vi "time_to_mass.vi"(1 "C1 Data":T3, 3 "C2 Data":T3, 5 "Vairables Cluster":T1, 11 "error in (no error)":errorcluster) -> (12 "C1 Mass Data":T2, 14 "C2 Mass Data":T2, 15 "error out":errorcluster)   [LabVIEW 2023]
uses:
  <vilib>/Waveform/WDTOps.llb/WDT Get Waveform Time Array DBL.vi
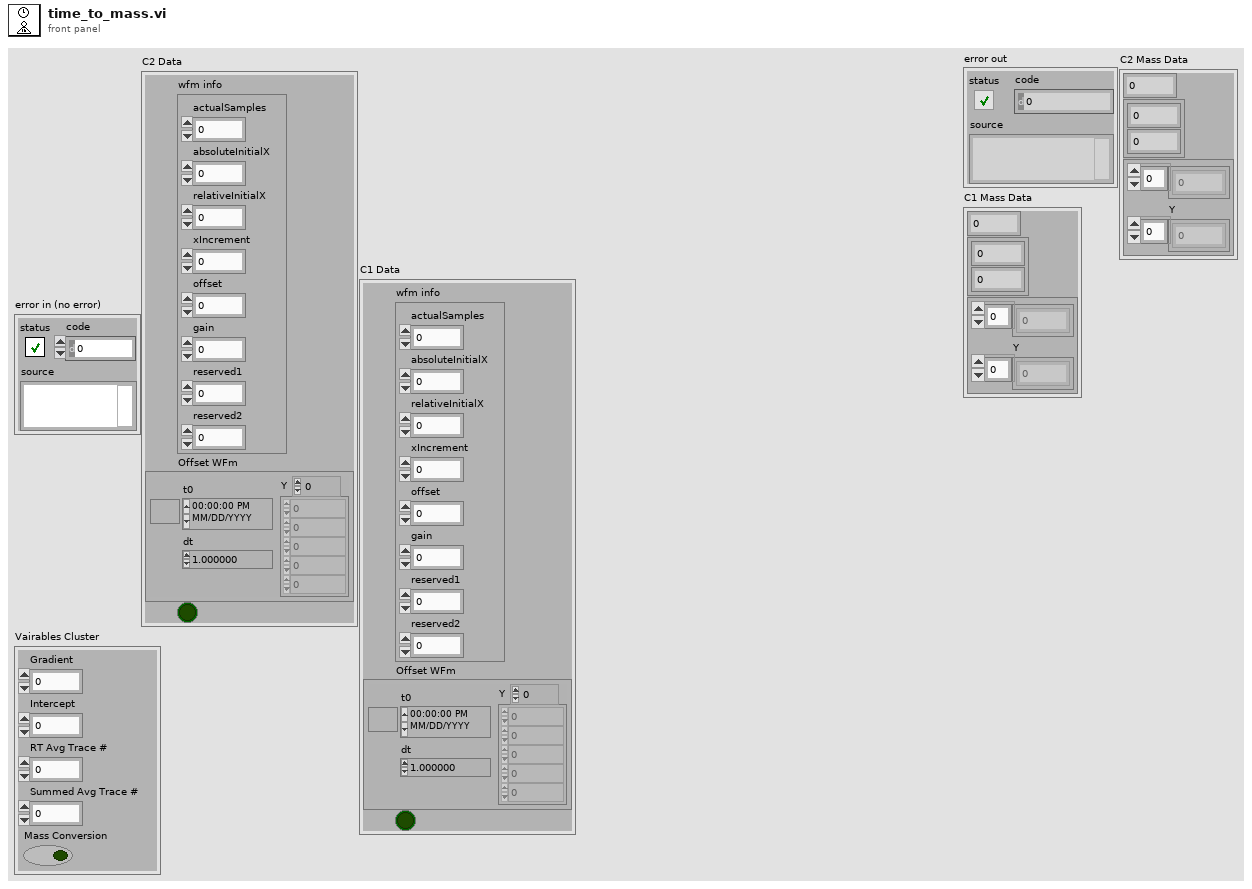
[diagram p1: front panel]
types:
  T1 = cluster{"Gradient":dbl, "Intercept":dbl, "RT Avg Trace #":i32, "Summed Avg Trace #":i32, "Mass Conversion":bool}
  T2 = cluster{dbl, cluster{dbl, dbl}, cluster{dbl[], "Y":dbl[]}}
  T3 = cluster{"wfm info":cluster{"actualSamples":i32, "absoluteInitialX":dbl, "relativeInitialX":dbl, "xIncrement":dbl, "offset":dbl, "gain":dbl, "reserved1":dbl, "reserved2":dbl}, "Offset WFm":waveform(dbl), bool}
  T4 = cluster{"actualSamples":i32, "absoluteInitialX":dbl, "relativeInitialX":dbl, "xIncrement":dbl, "offset":dbl, "gain":dbl, "reserved1":dbl, "reserved2":dbl}
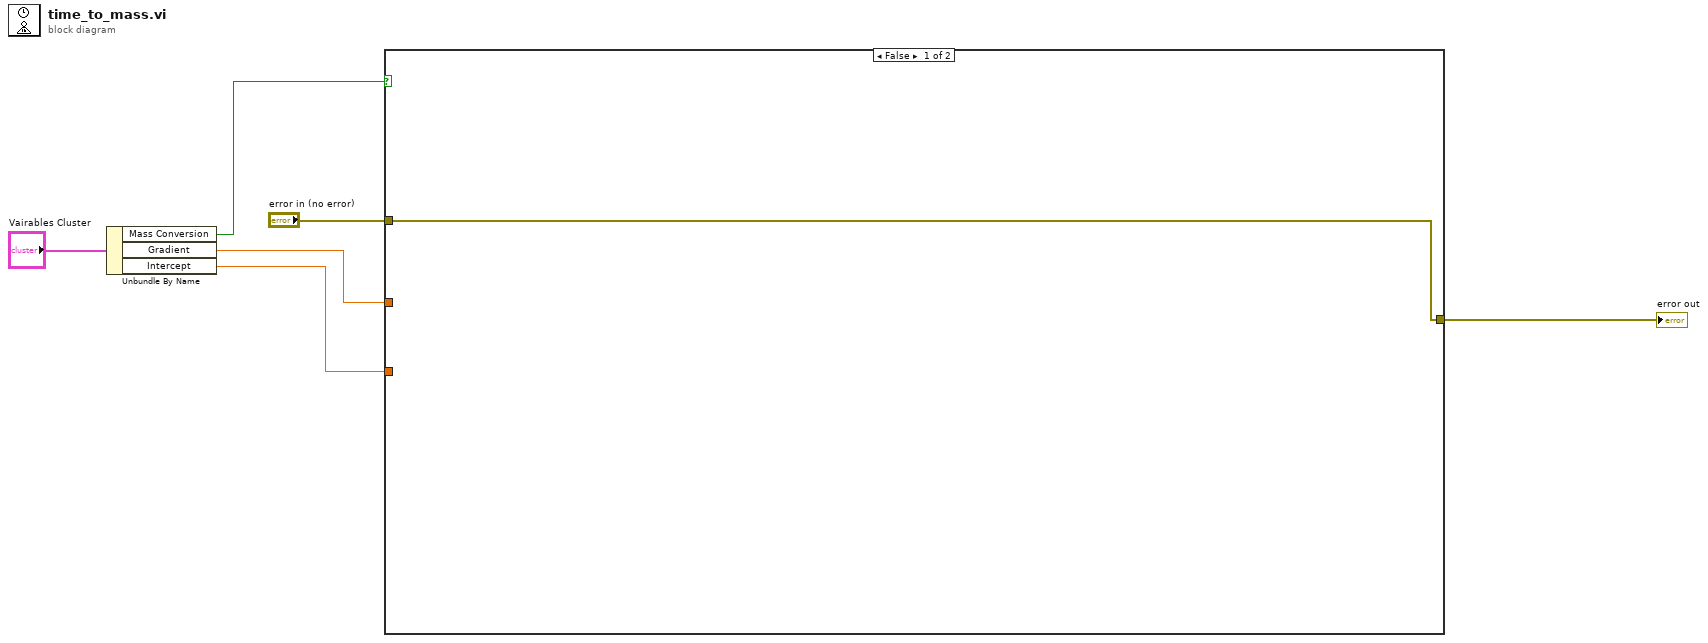
[diagram p0: block diagram]
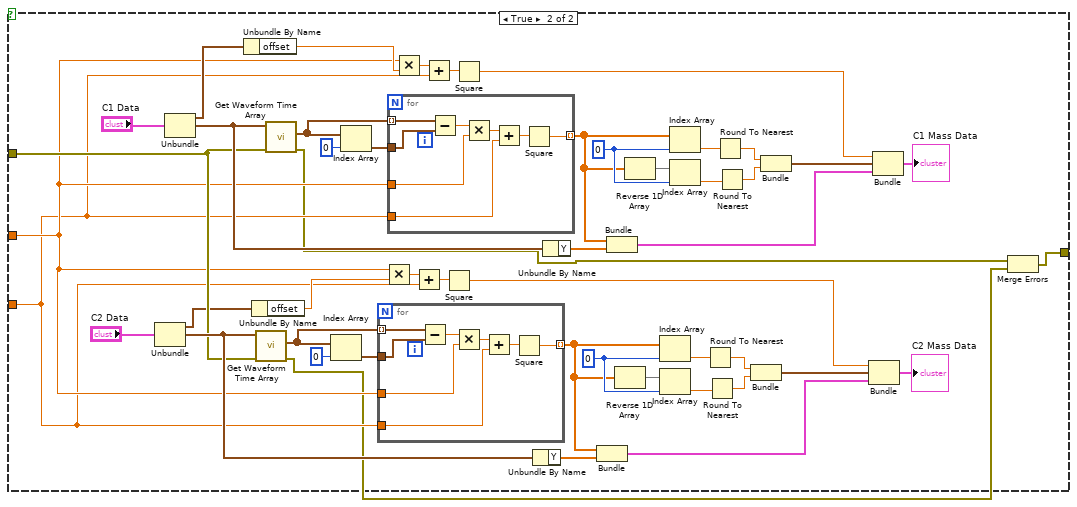
[diagram p2: hidden frame]
diagram:
  n1 = Unbundle By Name("Vairables Cluster") -> ("Mass Conversion"=w3:bool, "Gradient"=w2:dbl, "Intercept"=w1:dbl)
  n2 = case shown="False" w3 {
    tunnel: "error in (no error)" -> [w7 w21]
    tunnel: w2 -> [_ w12]
    tunnel: w1 -> [_ w11]
    tunnel: [w7 w8] -> w5
    frame False {
    }
    frame True {
      w32 = 0 ("index")
      w49 = 0 ("index")
      n3 = Unbundle("C2 Data") -> ("wfm info"=w16:T4, "Offset WFm"=w27:waveform(dbl))  [unwired: 1 out]
      n4 = Unbundle("C1 Data") -> ("wfm info"=w18:T4, "Offset WFm"=w44:waveform(dbl))  [unwired: 1 out]
      n5 = Unbundle By Name(w18) -> ("offset"=w17:dbl)
      n6 = Unbundle By Name(w16) -> ("offset"=w15:dbl)
      n7 = call-poly <vilib>:"Get Waveform Time Array.vi"("error in (no error)"=w21, "waveform in"=w27) -> ("error out"=w9:errorcluster, "X array"=w36:timestamp[])  [unwired: 8 in]
      n8 = call-poly <vilib>:"Get Waveform Time Array.vi"("error in (no error)"=w21, "waveform in"=w44) -> ("error out"=w10:errorcluster, "X array"=w53:timestamp[])  [unwired: 8 in]
      n9 = Index Array(array=w36, index=0) -> (element=w37:timestamp)
      n10 = Index Array(array=w53, index=0) -> (element=w54:timestamp)
      n11 = for {
        tunnel: w37 -> [w62]
        tunnel: w36 -> [w63] mode=indexing
        tunnel: w11 -> [w60]
        tunnel: [w58] -> w25 mode=indexing
        tunnel: w12 -> [w56]
        n12 = Subtract(x=w63, y=w62) -> (x-y=w57:dbl)
        n13 = Multiply(x=w57, y=w56) -> (x*y=w61:dbl)
        n14 = Add(x=w61, y=w60) -> (x+y=w59:dbl)
        n15 = Square(x=w59) -> (x^2=w58:dbl)
      }
      n16 = Multiply(x=w12, y=w15) -> (x*y=w35:dbl)
      n17 = for {
        tunnel: w54 -> [w70]
        tunnel: w53 -> [w71] mode=indexing
        tunnel: w11 -> [w68]
        tunnel: [w66] -> w42 mode=indexing
        tunnel: w12 -> [w64]
        n18 = Subtract(x=w71, y=w70) -> (x-y=w65:dbl)
        n19 = Multiply(x=w65, y=w64) -> (x*y=w69:dbl)
        n20 = Add(x=w69, y=w68) -> (x+y=w67:dbl)
        n21 = Square(x=w67) -> (x^2=w66:dbl)
      }
      n22 = Multiply(x=w12, y=w17) -> (x*y=w52:dbl)
      n23 = Add(x=w35, y=w11) -> (x+y=w34:dbl)
      n24 = Add(x=w52, y=w11) -> (x+y=w51:dbl)
      n25 = Square(x=w34) -> (x^2=w22:dbl)
      n26 = Square(x=w51) -> (x^2=w39:dbl)
      n27 = Unbundle By Name(w27) -> ("Y"=w26:dbl[])
      n28 = Unbundle By Name(w44) -> ("Y"=w43:dbl[])
      n29 = Bundle(w25, "Y"=w26) -> (w24:cluster{dbl[], "Y":dbl[]})  [unwired: 1 in]
      n30 = Bundle(w42, "Y"=w43) -> (w41:cluster{dbl[], "Y":dbl[]})  [unwired: 1 in]
      n31 = Reverse 1D Array(array=w25) -> (reversed array=w33:dbl[])
      n32 = Reverse 1D Array(array=w42) -> (reversed array=w50:dbl[])
      n33 = Index Array(array=w25, index=w32) -> (element=w31:dbl)
      n34 = Index Array(array=w33, index=w32) -> (element=w30:dbl)
      n35 = Index Array(array=w42, index=w49) -> (element=w48:dbl)
      n36 = Index Array(array=w50, index=w49) -> (element=w47:dbl)
      n37 = Round To Nearest(number=w31) -> (nearest integer value=w29:dbl)
      n38 = Round To Nearest(number=w30) -> (nearest integer value=w28:dbl)
      n39 = Round To Nearest(number=w48) -> (nearest integer value=w46:dbl)
      n40 = Round To Nearest(number=w47) -> (nearest integer value=w45:dbl)
      n41 = Bundle(w29, w28) -> (w23:cluster{dbl, dbl})  [unwired: 1 in]
      n42 = Bundle(w46, w45) -> (w40:cluster{dbl, dbl})  [unwired: 1 in]
      n43 = Bundle(w22, w23, w24) -> (→"C2 Mass Data":T2)  [unwired: 1 in]
      n44 = Bundle(w39, w40, w41) -> (→"C1 Mass Data":T2)  [unwired: 1 in]
      n45 = Merge Errors(w10, w9) -> (w8:errorcluster)
    }
  }
  "error out" <- w5
